vi "HAL camera get one frame.vi"(2 "error in":errorcluster, 3 "New Image":T1, 4 "Camera Parameters (important)":T2={"Exposure Time (sec)"=0.0, "EM CCD Gain"=0, "Readout Settings"={"Clocking mode"=1, "Speed"=3, "Clear mode"=2, "# clear cycles"=2, "ADC Gain"=2}, "Image Size"={"H Bin"=1, "V Bin"=1, "Left"=1, "Top"=1, "Right"=512, "Bottom"=512}} {"Readout Settings"."ADC Gain" min=-1 step=1; "Readout Settings"."Clear mode" items=["Don't clear", "Clear pre-exposure", "Clear pre-sequence", "Clear post-sequence", "Clear pre- and post-sequence", "Clear pre-exposure and post-sequence"]; "Readout Settings"."Speed" items=["1 Mhz, no EM", "5 Mhz, no EM", "5 Mhz, EM", "10 MHz, EM"]; "Readout Settings"."Clocking mode" items=["Normal", "Frame-transfer"]; "EM CCD Gain" scale=0.01..4096.0; "Exposure Time (sec)" scale=0.001..10.0 scale format="%#_1g"}) -> (0 "error out":errorcluster, 1 "Image Out":T1)   [LabVIEW 2011]
uses:
  Cascade-specific globals.vi
  <vilib>/vision/Image Controls.llb/IMAQ Image.ctl
  Camera/Image size.ctt
  cascade readout settings.ctl
  HAL camera parameters important.ctt
panel:
  # "Camera: Roper Cascade"
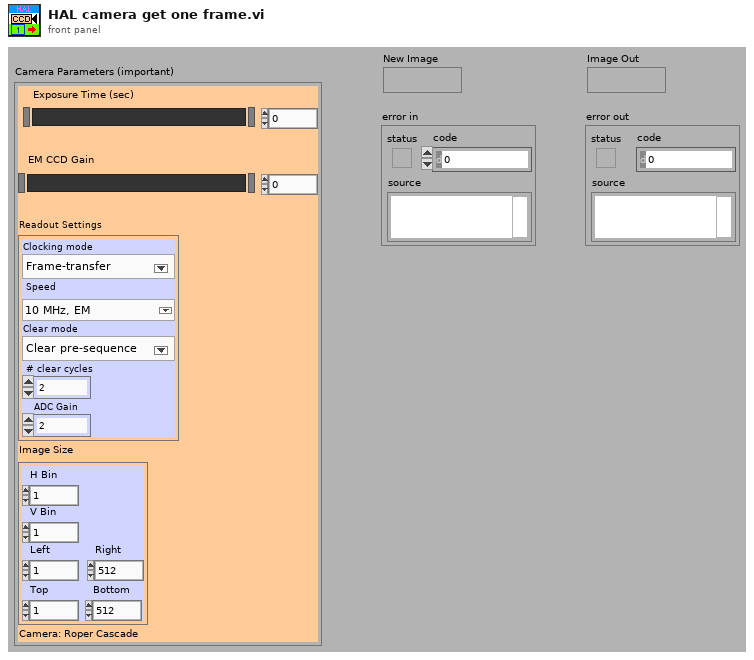
[diagram p1: front panel]
types:
  T1 = typedef "IMAQ Image.ctl" = refnum<image>
  T2 = typedef "HAL camera parameters important.ctt" = cluster{"Exposure Time (sec)":sgl, "EM CCD Gain":u16, "Readout Settings":T3, "Image Size":T4}
  T3 = typedef "cascade readout settings.ctl" = cluster{"Clocking mode":u8, "Speed":u16, "Clear mode":u8, "# clear cycles":u16, "ADC Gain":i32}
  T4 = typedef "Image size.ctt" = cluster{"H Bin":i32, "V Bin":i32, "Left":i32, "Top":i32, "Right":i32, "Bottom":i32}
  T5 = cluster{"Camera Handle":u32, "Pulser Handle":u32, "File Handle":u32, "Display Handle":u32, "Image Handle":u32}
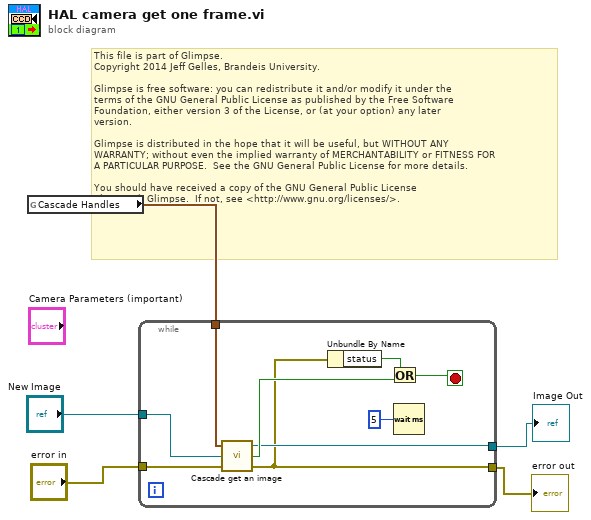
[diagram p0: block diagram]
diagram:
  # "This file is part of Glimpse. \nCopyright 2014 Jeff Gelles, Brandeis University.    \n\nGlimpse is free software: you can redistribute it and/or modify it under the \nterms of the GNU General Public License as published by the Free Software \nFoundation, either version 3 of the License, or (at your option) any later \nversion.\n\nGlimpse is distributed in the hope that it will be useful, but WITHOUT ANY \nWARRANTY; without even the implied warranty of MERCHANTABILITY or FITNESS FOR \nA PARTICULAR PURPOSE.  See the GNU General Public License for more details.\n\nYou should have received a copy of the GNU General Public License\nalong with Glimpse.  If not, see <http://www.gnu.org/licenses/>."
  n1 = global read "Cascade-specific globals.vi" "Cascade Handles"() -> (w3:T5)
  n2 = while {
    tunnel: [w12] -> w2
    tunnel: [w11] -> w1
    tunnel: "error in" -> [w8]
    tunnel: "New Image" -> [w7]
    tunnel: w3 -> [w6]
    stop <- w13 stop-if-true
    n3 = call "Cascade get an image.vi"("error in"=w8, "Image In"=w7, "Handles in"=w6) -> ("error out"=w11:errorcluster, "new image acquired?"=w14:bool, "Image Out"=w12:T1)
    n4 = Unbundle By Name(w11) -> ("status"=w9:bool)
    n5 = Or(x=w9, y=w14) -> (x .or. y?=w13:bool)
    n6 = Wait (ms)(milliseconds to wait=u32 5) -> ()  [unwired: 1 out]
  }
  "Image Out" <- w2
  "error out" <- w1
